vi "WriteConnInfo.vi"(8 "error in (no error)":errorcluster, 11 "connection info":T1) -> (0 "error out":errorcluster)   [LabVIEW 2017, in "ServerComm.lvlib"]
uses:
  <vilib>/addons/InsightCM/Devices/Shared/Common/ServerComm/ServerComm.lvlib
  <vilib>/addons/InsightCM/MessageBus/Base/controls/ConnectionInfo.ctl
  <vilib>/addons/InsightCM/Utilities/GlobalConfiguration/GlobalConfiguration.lvlib
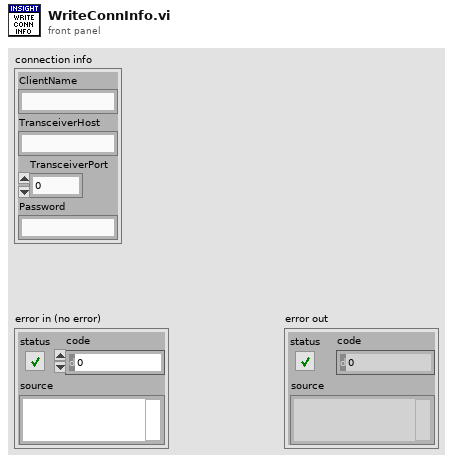
[diagram p1: front panel]
types:
  T1 = typedef "ConnectionInfo.ctl" = cluster{"ClientName":string, "TransceiverHost":string, "TransceiverPort":u16, "Password":string}
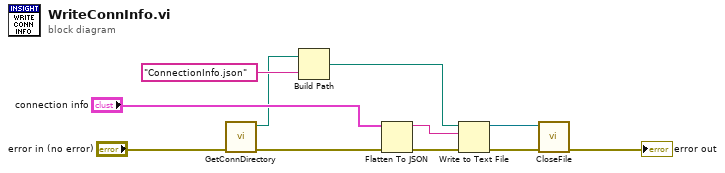
[diagram p0: block diagram]
diagram:
  n1 = call <vilib>:"GetConnDirectory.vi"("error in (no error)"="error in (no error)") -> ("error out"=w5:errorcluster, "application directory"=w4:path)  [unwired: 9 in]
  n2 = Build Path(base path=w4, name or relative path="ConnectionInfo.json") -> (appended path=w8:path)
  n3 = Flatten To JSON(anything="connection info", error in (no error)=w5) -> (JSON string=w7:string, 11:w10:errorcluster)  [unwired: 1 in]
  n4 = Write to Text File(file (use dialog)=w8, text=w7, error in=w10) -> (refnum out=w3:refnum<file>, error out=w2:errorcluster)  [unwired: 1 in, 1 out]
  n5 = call <vilib>:"CloseFile.vi"("error in (no error)"=w2, "file reference"=w3) -> ("error out"=→"error out":errorcluster)  [unwired: 9 in]
